vi "LoadAndRun.vi"(3 "error in (no error)":errorcluster, 4 "run?":bool, 5 "path":path) -> (0 "error out":errorcluster, 2 "vi refnum out":refnum<vi>)   [LabVIEW 2012]
doc: "Opens a refnum to the specified VI and, optionally, runs it."
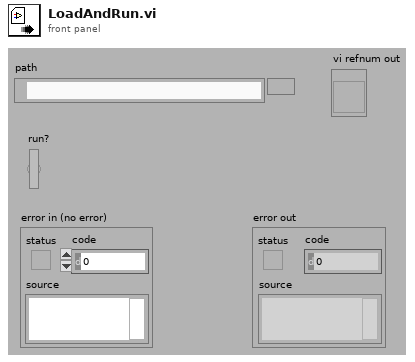
[diagram p1: front panel]
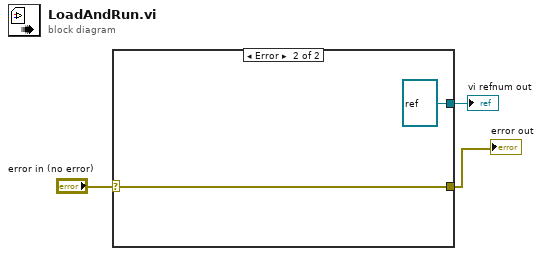
[diagram p0: block diagram]
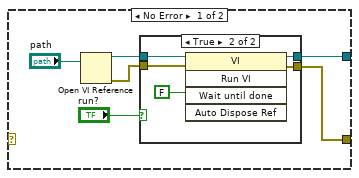
[diagram p2: hidden frame]
diagram:
  n1 = case shown="Error" "error in (no error)" {
    selector: "error in (no error)" -> [_ w17]
    tunnel: [w6 refnum<vi> refnum] -> w2
    tunnel: [w4 w17] -> w1
    frame No Error {
      n2 = Open VI Reference(vi path="path") -> (vi reference=w7:refnum<vi>, error out=w5:errorcluster)  [unwired: 5 in]
      n3 = case shown="True" "run?" {
        tunnel: w7 -> [w11 w16]
        tunnel: [w11 w14] -> w6
        tunnel: w5 -> [w10 w13]
        tunnel: [w10 w12] -> w4
        frame False {
        }
        frame True {
          n4 = invoke class="VI" method="Run VI"(reference=w16, error in=w13, "Wait until done"=FALSE) -> (reference out=w14:refnum<vi>, error out=w12:errorcluster)  [unwired: 2 in, 3 out]
        }
      }
    }
    frame Error {
    }
  }
  "vi refnum out" <- w2
  "error out" <- w1
